vi "Parse-Hex-String-to-U8.vi"() -> ()   [LabVIEW 2018]
uses:
  <userlib>/_OpenG.lib/string/string.llb/Trim Whitespace (String)__ogtk.vi
panel:
  out "Ethernet Frame\n(u8 [])":u32[](array[numeric]) format="%.0x"
  in  "String":string
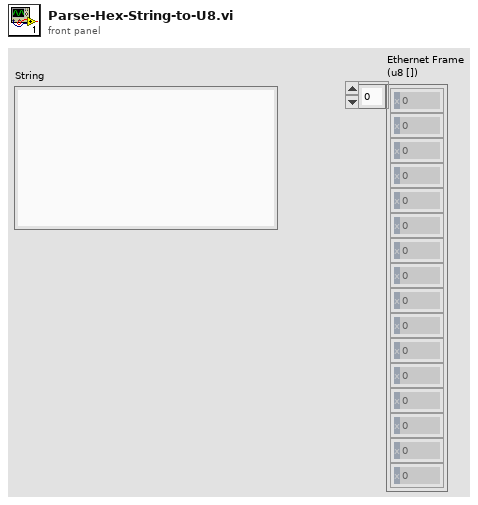
[diagram p1: front panel]
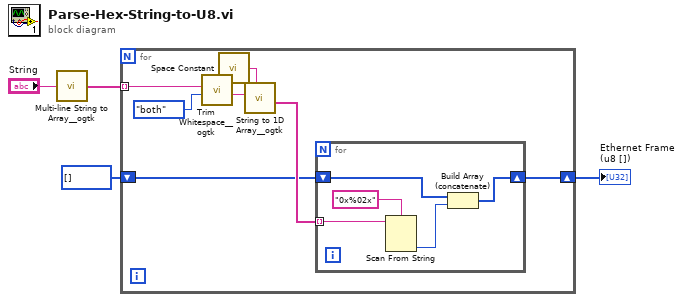
[diagram p0: block diagram]
diagram:
  n1 = call <userlib>:"Multi-line String to Array__ogtk.vi"("string"="String") -> ("lines"=w3:string[])
  n2 = for {
    tunnel: w3 -> [w11] mode=indexing
    shift-right: [w6] -> w2
    shift-left: u32[] [] -> [w5]
    n3 = call-poly <userlib>:"Trim Whitespace__ogtk.vi"("Remove (leading and trailing)"=enum16{"leading", "trailing", "both"}."both", "String in"=w11) -> ("String out"=w8:string)  [unwired: 5 in]
    n4 = call <vilib>:"Space Constant.vi"() -> ("String"=w9:string)
    n5 = call <userlib>:"String to 1D Array__ogtk.vi"("delimiter (Tab)"=w9, "string"=w8) -> ("Array of Strings"=w7:string[])  [unwired: 9 in]
    n6 = for {
      tunnel: w7 -> [w16] mode=indexing
      shift-right: [w13] -> w6
      shift-left: w5 -> [w12]
      n7 = Scan From String(format string="0x%02x", input string=w16) -> (output 1=w14:u32)  [unwired: 3 in, 3 out]
      n8 = Build Array (concatenate)(w12, w14) -> (w13:u32[])
    }
  }
  "Ethernet Frame\n(u8 [])" <- w2
